vi "Selection_Prompt.vi"(8 "error in (no error)":errorcluster) -> (0 "error out":errorcluster, 2 "OK":bool, 3 "Collect Data":bool)   [LabVIEW 2018]
doc: "This VI prompts the user to select a method to calculate the acceleration due to gravity. It can either run a test or open a data file.\n\nInputs:\nError in.\n\nOutputs:\nError out;\nOK;\nCollect Data."
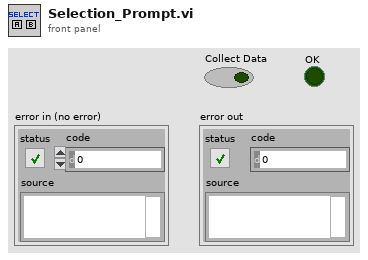
[diagram p1: front panel]
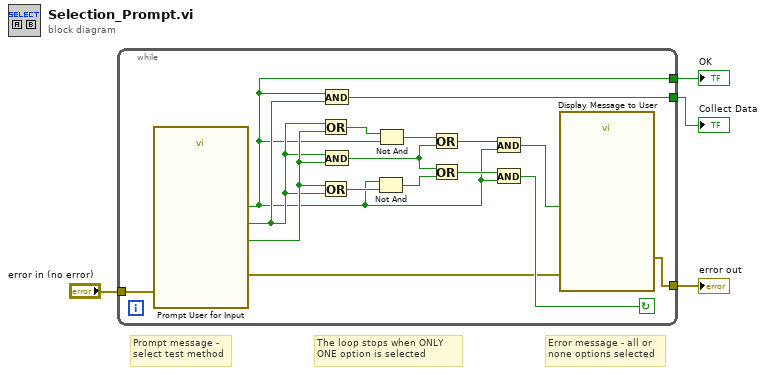
[diagram p0: block diagram]
diagram:
  # "The loop stops when ONLY\nONE option is selected"
  # "Error message - all or\nnone options selected"
  # "Prompt message -\nselect test method"
  n1 = while {
    tunnel: "error in (no error)" -> [w20]
    tunnel: [w6] -> w3
    tunnel: [w12] -> w4
    tunnel: [w5] -> w1
    stop <- w8 continue-if-true
    n2 = call "Prompt User for Input"("error in (no error)"=w20) -> ("Open Data File"=w15:bool, "Run Test"=w13:bool, "OK"=w5:bool, "error out"=w7:errorcluster)  [unwired: 15 in]
    n3 = Or(x=w13, y=w15) -> (x .or. y?=w14:bool)
    n4 = Or(x=w15, y=w13) -> (x .or. y?=w16:bool)
    n5 = And(x=w5, y=w13) -> (x .and. y?=w12:bool)
    n6 = And(x=w13, y=w15) -> (x .and. y?=w19:bool)
    n7 = Not And(1:w16, 2:w5) -> (0:w18:bool)
    n8 = Not And(1:w5, 2:w14) -> (0:w17:bool)
    n9 = Or(x=w17, y=w19) -> (x .or. y?=w10:bool)
    n10 = Or(x=w19, y=w18) -> (x .or. y?=w11:bool)
    n11 = And(x=w10, y=w5) -> (x .and. y?=w9:bool)
    n12 = And(x=w11, y=w5) -> (x .and. y?=w8:bool)
    n13 = call "Display Message to User"("error in (no error)"=w7, "Enable"=w9) -> ("error out"=w6:errorcluster)  [unwired: 8 in, 1 out]
  }
  "Collect Data" <- w4
  "error out" <- w3
  "OK" <- w1
